vi "Main.vi"(8 "error in (no error)":errorcluster, 11 "DAQMH121119OrcaFlashBase in":refnum<class "DAQOrcaFlash.lvclass">) -> (0 "error out":errorcluster, 3 "component":refnum<class "DAQOrcaFlash.lvclass">)   [LabVIEW 2012, in "DAQOrcaFlash.lvclass"]
doc: "Main VI of the component."
uses:
  DAQOrcaFlash.lvclass
  binning.ctl
  visualisation_line_cluster.ctl
  merit_factor_type.ctl
  DAQOrcaFlash.lvclass/DAQOrcaFlash.ctl
  <vilib>/Distrio/Murmex/InitialiseMessage/InitialiseMessage.lvclass
  <vilib>/Distrio/Murmex/Murmex/command_enum.ctl
  <vilib>/Distrio/Murmex/TerminateMessage/TerminateMessage.lvclass
  <vilib>/Distrio/Murmex/StartMessage/StartMessage.lvclass
  <vilib>/Distrio/Murmex/StartMessage/run mode enum.ctl
  <vilib>/Distrio/Murmex/StopMessage/StopMessage.lvclass
  <vilib>/Distrio/Murmex/ConfigureMessage/ConfigureMessage.lvclass
  <vilib>/Distrio/Murmex/Murmex/update_cluster.ctl
  class variable.vi
  <vilib>/Distrio/Murmex/Murmex/Set VI reference.vi
  <vilib>/Distrio/Murmex/Murmex/Set configure at initialise.vi
  <vilib>/Distrio/Murmex/Murmex/Set relay start stop to observers.vi
  <vilib>/Distrio/Murmex/Murmex/Set log reference.vi
  <vilib>/Distrio/Murmex/Murmex/Set write log to disk.vi
  <vilib>/Distrio/Murmex/Murmex/Murmex.lvclass
  <vilib>/Distrio/Murmex/Message/Message.lvclass
panel:
  in  "button:configure":bool
  in  "button:quit":bool
  in  "terminate?":bool
  out "progress bar":sgl(slide) scale=0.0..1.0
  in  "Tab":T1(tab)
  in  "Rolling shutter pace":sgl[unit]=9.74436e-06 min=9.74436e-06 max=10 step=3.76e-09 format="%#_7g"
  out "Frames per second":dbl[unit]
  out "Virtual slit width":dbl[unit]
  in  "button:start_sweep":bool
  in  "y offset":u16 max=2048 step=4
  in  "x offset":u16 max=2048 step=4
  in  "y resolution":u16=2048 min=4 max=2048 step=4
  in  "x resolution":u16=2048 min=4 max=2048 step=4
  in  "binning":T2=1 items=["1x1"=1, "2x2"=2, "4x4"=4]
  in  "no. of frames":i32=1 min=1 step=1
  in  "line exposure time":dbl[unit]=0.1 caption="exposure time" min=9.700000000000001e-09 max=0.01
  in  "button:start focus":bool
  in  "file name":string
  in  "subfolder levels":string[](array[string])
  in  "Custom saving path":bool
  in  "directory out":path
  in  "button:convert":bool
  out "filename":string
  in  "directory in":path
  in  "ID":string="orca"
  in  "log":string
  out "time interval between MF":dbl
  out "Merit Factor":dbl
  in  "Merit factor type":T3
  in  "button:AO":bool
  in  "lines":T4[](array[typedef])
  in  "Conversion policy":T5={"Conversion Method"=10, "Minimum Value"=0, "Maximum Value"=0, "# Shifts"=0} {"Conversion Method" items=["Default"=10, "Most Significant Bits"=11, "Full Dynamic"=12, "Downshift"=13, "Given Range"=14, "90% Dynamic"=15, "Given Percent Range"=16]}
  # "Convert here properietary file formats of Hamamatsu to TIFF format."
  # "DAQOrcaFlash\n\nImplemented by:\nMarcel van 't Hoff\nLudovico Silvestri\nUniversity of Florence, Ital\n\nThis component supports only the Hamamatsu Orca Flash 4.0"
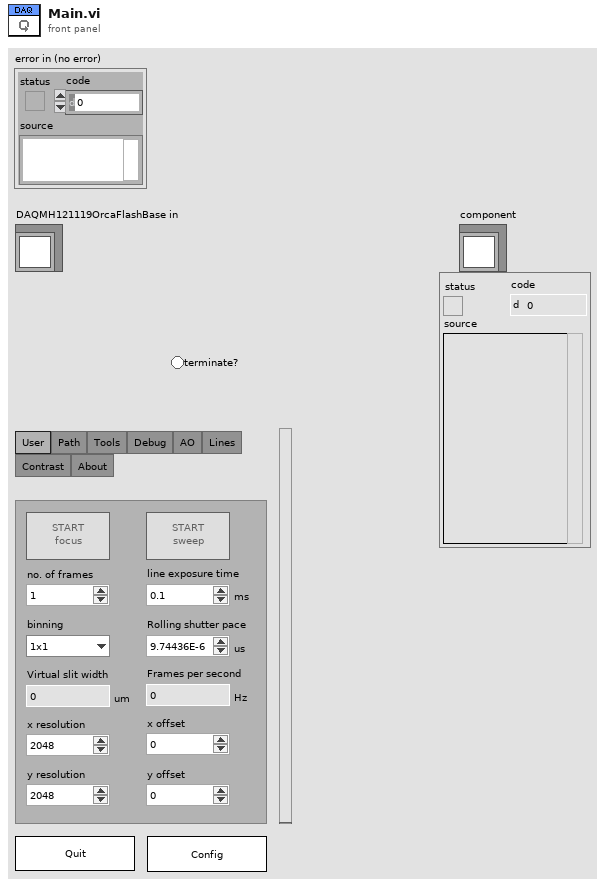
[diagram p1: front panel]
types:
  T1 = enum32{"User", "Path", "Tools", "Debug", "AO", "Lines", "Contrast", "About"}
  T2 = typedef "DAQOrcaFlash.lvclass/binning.ctl" = u16
  T3 = typedef "DAQOrcaFlash.lvclass/merit_factor_type.ctl" = enum16{"full frame intensity", "ROI beads", "Weber contrast", "Michelson contrast", "RMS contrast", "Line profile analysis", "ROI analysis", "FFT", "SNR", "5% brightest"}
  T4 = typedef "DAQOrcaFlash.lvclass/visualisation_line_cluster.ctl" = cluster{"direction":enum16{"horizontal", "vertical"}, "position":i32}
  T5 = cluster{"Conversion Method":u32, "Minimum Value":i32, "Maximum Value":i32, "# Shifts":i32}
  T6 = typedef "Murmex.lvlib/Murmex.lvclass/command_enum.ctl" = enum16{"null", "initialise", "reset", "terminate", "acknowledge", "update", "inspect", "inform", "proceed", "start", "stop", "fetch", "configure", "generic"}
  T7 = typedef "Murmex.lvlib/StartMessage.lvclass/run mode enum.ctl" = enum16{"infinite", "finite"}
  T8 = typedef "Murmex.lvlib/Murmex.lvclass/update_cluster.ctl" = cluster{"target ID":string, "key chains":string[], "values":variant[]}
  T9 = enum8{"Enabled", "Disabled", "Disabled and Grayed Out"}
  T10 = typedef "Murmex.lvclass/command_enum.ctl" = enum16{"null", "initialise", "reset", "terminate", "acknowledge", "update", "inspect", "inform", "proceed", "start", "stop", "fetch", "configure", "generic"}
  T11 = typedef "Murmex.lvclass/Event type enumerations.ctl" = enum16{"before", "after"}
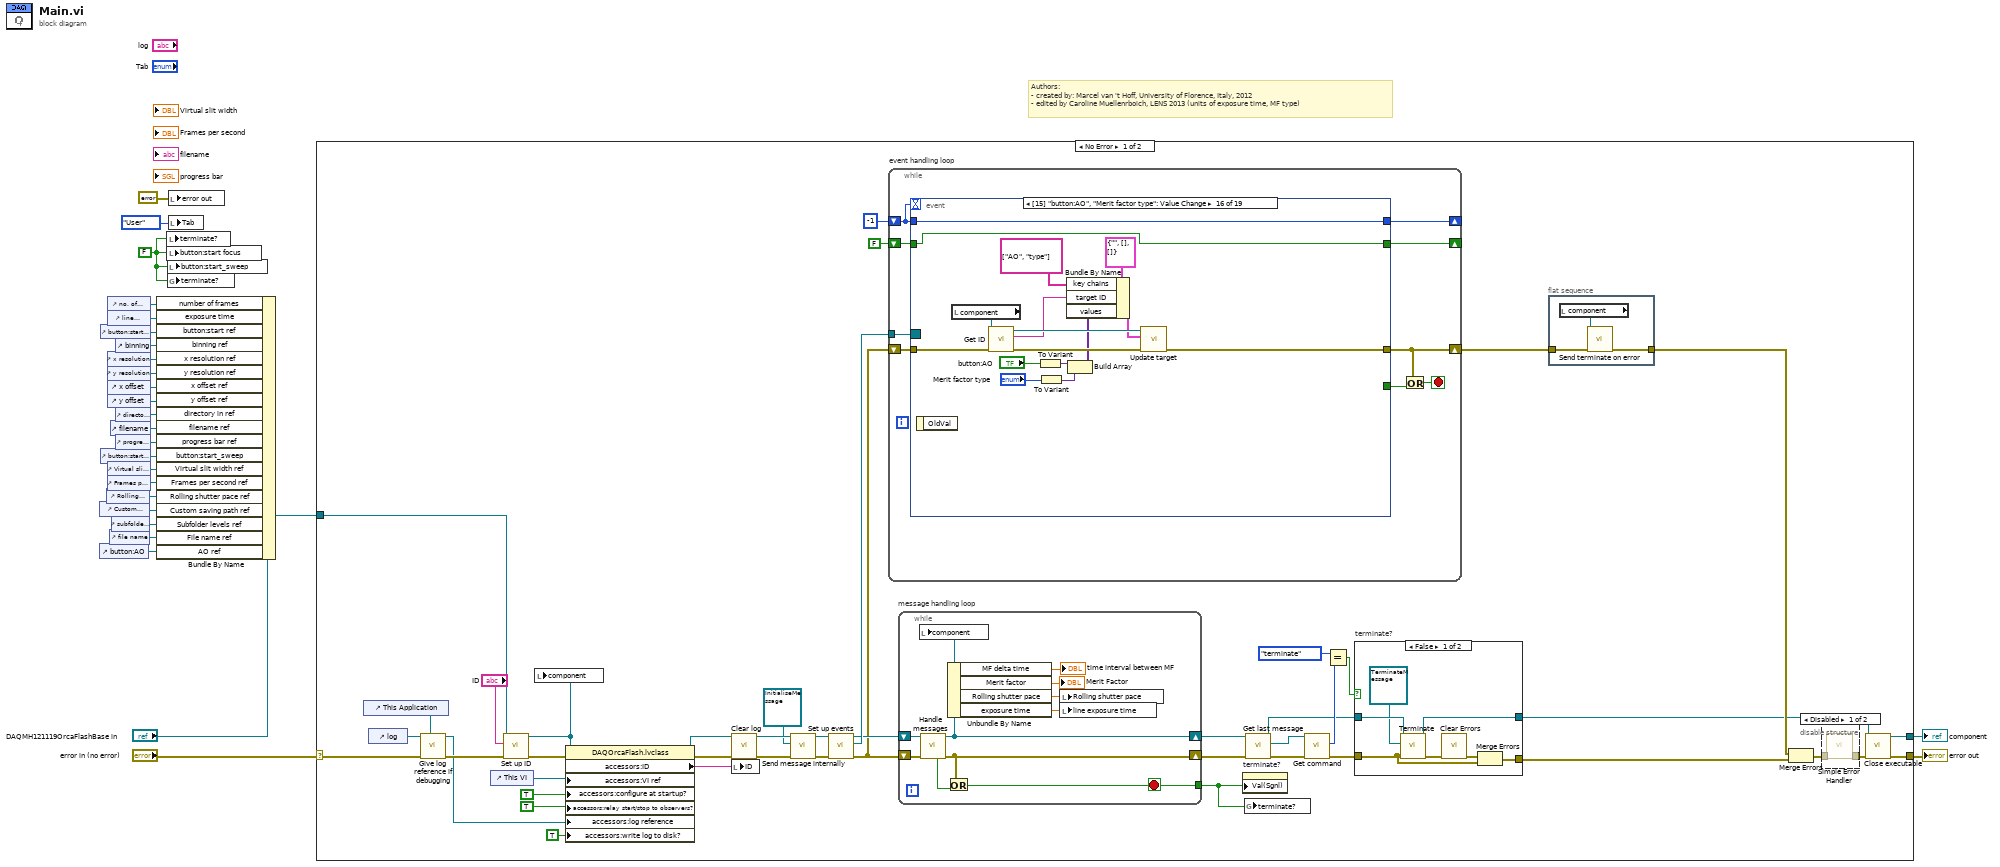
[diagram p0: block diagram]
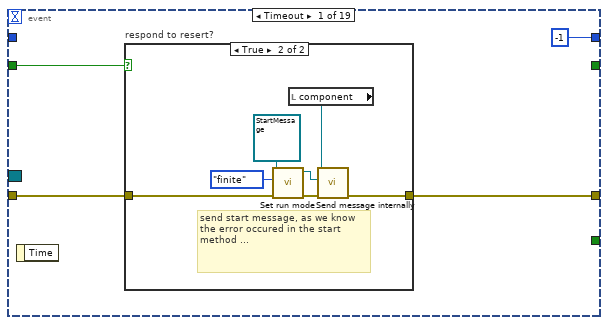
[diagram p4: hidden frame]
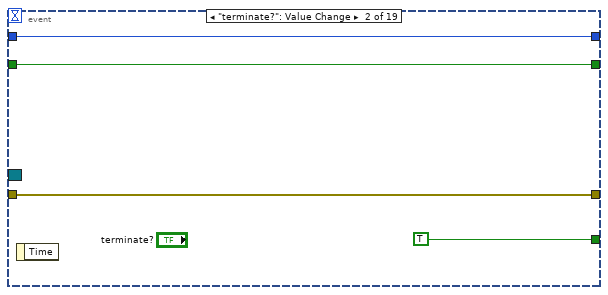
[diagram p6: hidden frame]
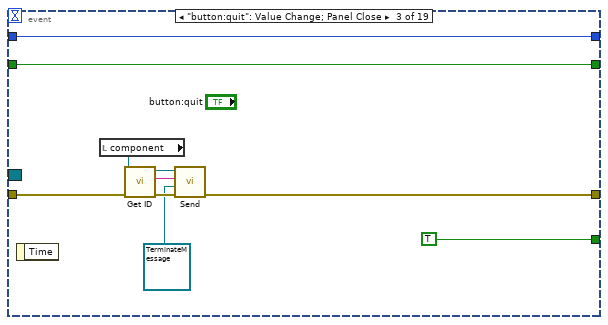
[diagram p7: hidden frame]
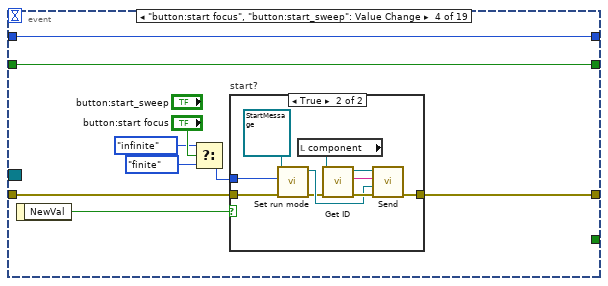
[diagram p8: hidden frame]
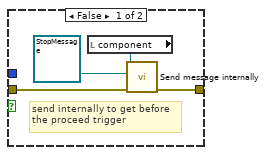
[diagram p9: hidden frame]
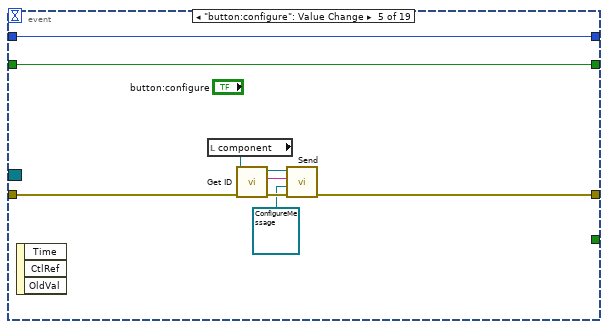
[diagram p10: hidden frame]
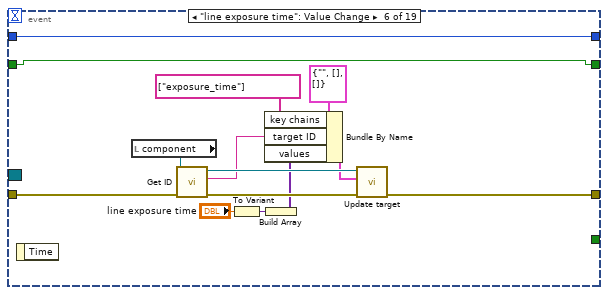
[diagram p11: hidden frame]
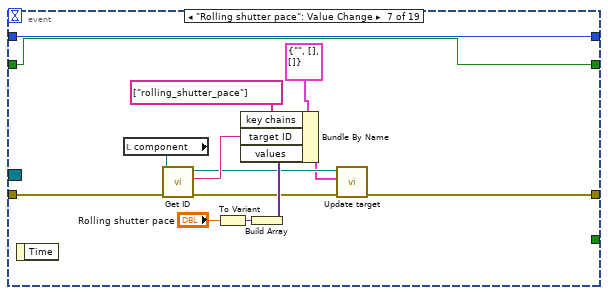
[diagram p12: hidden frame]
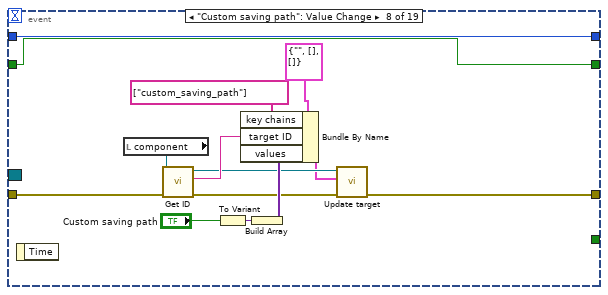
[diagram p13: hidden frame]
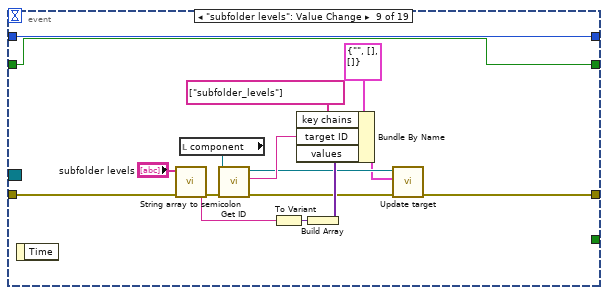
[diagram p14: hidden frame]
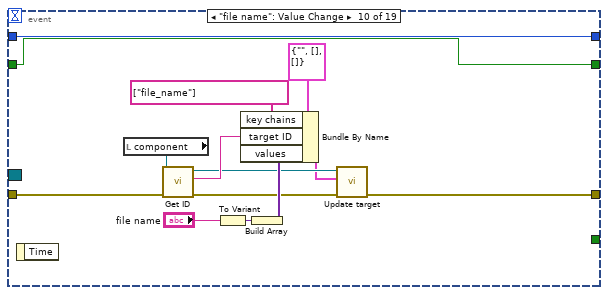
[diagram p15: hidden frame]
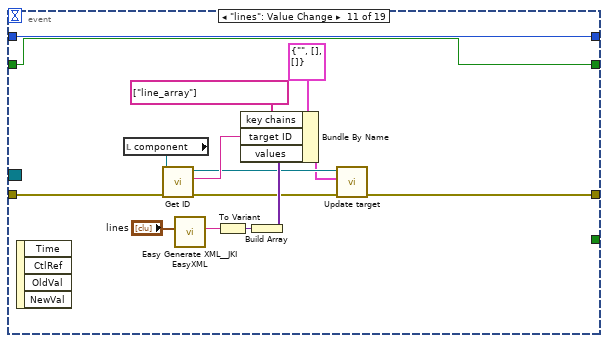
[diagram p16: hidden frame]
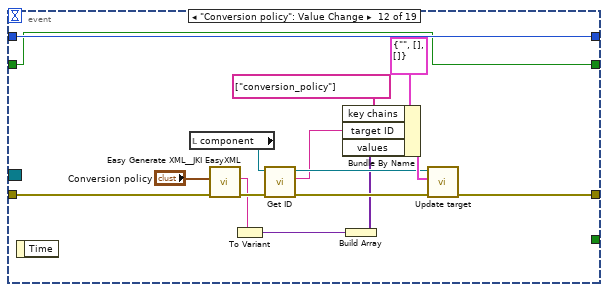
[diagram p17: hidden frame]
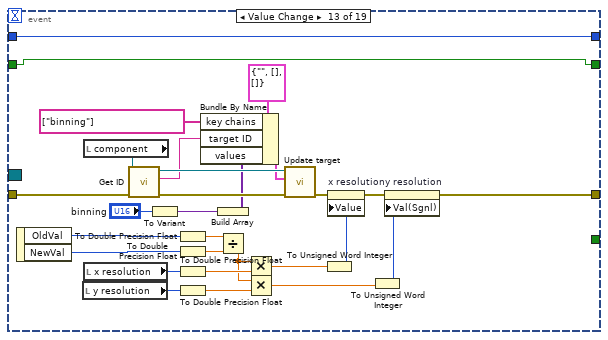
[diagram p18: hidden frame]
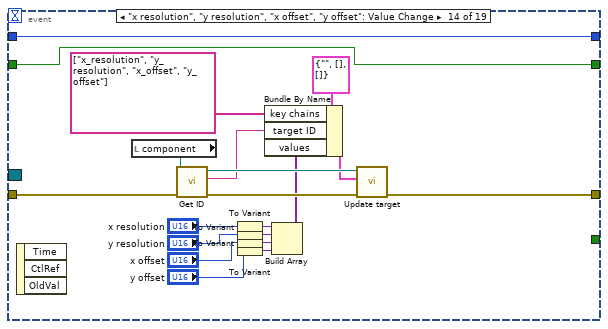
[diagram p19: hidden frame]
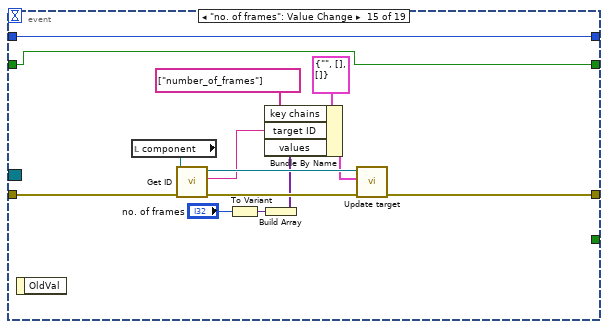
[diagram p20: hidden frame]
diagram:
  w9 = FALSE ("terminate?")
  # "Authors: \n- created by: Marcel van 't Hoff, University of Florence, Italy, 2012\n- edited by Caroline Muellenrboich, LENS 2013 (units of exposure time, MF type)"
  n1 = control-ref of="button:AO"() -> (w2:refnum<vi>)
  n2 = control-ref of="Custom saving path"() -> (w3:refnum<vi>)
  n3 = control-ref of="button:start focus"() -> (w20:refnum<vi>)
  n4 = control-ref of="button:start_sweep"() -> (w10:refnum<vi>)
  n5 = control-ref of="Rolling shutter pace"() -> (w6:refnum<vi>)
  n6 = control-ref of="no. of frames"() -> (w21:refnum<vi>)
  n7 = control-ref of="line exposure time"() -> (w22:refnum<vi>)
  n8 = control-ref of="x resolution"() -> (w18:refnum<vi>)
  n9 = control-ref of="y resolution"() -> (w17:refnum<vi>)
  n10 = control-ref of="x offset"() -> (w16:refnum<vi>)
  n11 = control-ref of="y offset"() -> (w15:refnum<vi>)
  n12 = control-ref of="Virtual slit width"() -> (w8:refnum<vi>)
  n13 = control-ref of="Frames per second"() -> (w7:refnum<vi>)
  n14 = control-ref of="file name"() -> (w5:refnum<vi>)
  n15 = control-ref of="filename"() -> (w13:refnum<vi>)
  n16 = control-ref of="subfolder levels"() -> (w4:refnum<vi>)
  n17 = control-ref of="binning"() -> (w19:refnum<vi>)
  n18 = control-ref of="directory in"() -> (w14:refnum<vi>)
  n19 = control-ref of="progress bar"() -> (w12:refnum<vi>)
  n20 = Bundle By Name(cluster="DAQMH121119OrcaFlashBase in", "number of frames"=w21, "exposure time"=w22, "button:start ref"=w20, "binning ref"=w19, "x resolution ref"=w18, "y resolution ref"=w17, "x offset ref"=w16, "y offset ref"=w15, "directory in ref"=w14, "filename ref"=w13, "progress bar ref"=w12, "button:start_sweep"=w10, "Virtual slit width ref"=w8, "Frames per second ref"=w7, "Rolling shutter pace ref"=w6, "Custom saving path ref"=w3, "Subfolder levels ref"=w4, "File name ref"=w5, "AO ref"=w2) -> (w23:refnum<class "DAQOrcaFlash.lvclass">)
  n21 = local write "terminate?"(w9) -> ()
  n22 = local write "button:start focus"(w9) -> ()
  n23 = local write "button:start_sweep"(w9) -> ()
  n24 = global write "class variable.vi" "terminate?"(w9) -> ()
  n25 = local write "error out"(errorcluster {"status"=FALSE, "code"=0, "source"=""} ("error out")) -> ()
  n26 = local write "Tab"(T1."User" ("Tab")) -> ()
  n27 = case shown="No Error" "error in (no error)" {
    selector: "error in (no error)" -> [w34 w423]
    tunnel: [w61 w423] -> w26
    tunnel: [w60 w422] -> w25
    tunnel: w23 -> [w66 w422]
    frame No Error {
      n28 = control-ref of="This Application"() -> (w30:refnum<vi>)
      n29 = control-ref of="log"() -> (w32:refnum<vi>)
      n30 = call "Give log reference if debugging.vi"("application ref"=w30, "error in (no error)"=w34, "log reference in"=w32) -> ("error out"=w33:errorcluster, "log reference out"=w31:refnum<vi>)  [unwired: 6 in, 1 out]
      n31 = control-ref of="This VI"() -> (w56:refnum<vi>)
      n32 = call <vilib>:"Set up ID.vi"("error in (no error)"=w33, "component ID"="ID", "MurmexBase in"=w66) -> ("error out"=w58:errorcluster, "MurmexBase out"=w47:refnum<class "DAQOrcaFlash.lvclass">)  [unwired: 6 in, 1 out]
      n33 = local write "component"(w47) -> ()
      n34 = property class="DAQOrcaFlash.lvclass"(reference=w47, error in=w58, "accessors:VI ref"=w56, "accessors:configure at startup?"=TRUE ("configure at startup?"), "accessors:relay start/stop to observers?"=TRUE ("relay start/stop to observers?"), "accessors:log reference"=w31, "accessors:write log to disk?"=TRUE ("write log to disk?")) -> (reference out=w54:refnum<class "DAQOrcaFlash.lvclass">, error out=w55:errorcluster, "accessors:ID"=w57:string)
      n35 = call <vilib>:"Clear log.vi"("error in (no error)"=w55, "MurmexBase in"=w54) -> ("error out"=w67:errorcluster, "MurmexBase out"=w71:refnum<class "DAQOrcaFlash.lvclass">)  [unwired: 8 in]
      n36 = local write "ID"(w57) -> ()
      n37 = call <vilib>:"Send message internally.vi"("error in (no error)"=w67, "Message"=refnum<class "InitialiseMessage.lvclass"> refnum ("Distrio Murmex 1.0:InitialiseMessage"), "Murmex in"=w71) -> ("error out"=w64:errorcluster, "Murmex out"=w63:refnum<class "DAQOrcaFlash.lvclass">)  [unwired: 7 in]
      n38 = call <vilib>:"Set up events.vi"("error in (no error)"=w64, "MurmexBase in"=w63) -> ("error out"=w36:errorcluster, "Event Registration Refnum"=w69:refnum<event-registration>, "MurmexBase out"=w38:refnum<class "DAQOrcaFlash.lvclass">)  [unwired: 7 in]
      n39 = while "event handling loop" {
        shift-right: [w95] -> _
        shift-left: -1 -> [w94]
        tunnel: w69 -> [w92]
        shift-right: [w91] -> w68
        shift-left: w36 -> [w93]
        shift-right: [w88] -> _
        shift-left: FALSE ("respond to reset?") -> [w87]
        stop <- w89 stop-if-true
        n40 = event shown="[15] \"button:AO\", \"Merit factor type\": Value Change" {
          selector: w92 -> [_ _ _ _ _ _ _ _ _ _ _ _ _ _ _ _ _ _ _]
          dyn-events: _ -> [_ _ _ _ _ _ _ _ _ _ _ _ _ _ _ _ _ _ _]
          timeout: w94 -> [_ _ _ _ _ _ _ _ _ _ _ _ _ _ _ _ _ _ _]
          tunnel: [-1 w111 w121 w130 w153 w167 w181 w195 w211 w225 w240 w256 w285 w305 w319 w335 w337 w399 w411] -> w95
          tunnel: w94 -> [_ w111 w121 w130 w153 w167 w181 w195 w211 w225 w240 w256 w285 w305 w319 w335 w342 w399 w411]
          tunnel: w93 -> [w97 w110 w114 w129 w149 w166 w180 w194 w200 w224 w239 w255 w284 w304 w318 w334 w343 w397 w408]
          tunnel: [w96 w110 w116 w128 w148 w165 w173 w183 w204 w217 w232 w250 w267 w303 w317 w323 w344 w396 w401] -> w91
          tunnel: [_ TRUE TRUE _ _ _ _ _ _ _ _ _ _ _ _ _ _ _ _] -> w90
          tunnel: [_ w108 w112 w122 w145 w154 w168 w182 w196 w212 w226 w241 w257 w286 w306 w322 w339 w393 w400] -> w88
          tunnel: w87 -> [w98 w108 w112 w122 w145 w154 w168 w182 w196 w212 w226 w241 w257 w286 w306 w322 w340 w393 w400]
          event Timeout {
            n41 = event-data() -> ()  [unwired: 1 in, 1 out]
            n42 = case "respond to resert?" shown="True" w98 {
              tunnel: w97 -> [w100 w103]
              tunnel: [w100 w107] -> w96
              frame False {
              }
              frame True {
                # "send start message, as we know the error occured in the start method ..."
                n43 = call <vilib>:"Set run mode.vi"("error in (no error)"=w103, "run mode"=run_mode_enum."finite", "StartMessage in"=refnum<class "StartMessage.lvclass"> refnum ("Distrio Murmex 1.0:StartMessage")) -> ("error out"=w102:errorcluster, "StartMessage out"=w104:refnum<class "StartMessage.lvclass">)  [unwired: 7 in]
                n44 = local read "component"() -> (w106:refnum<class "DAQOrcaFlash.lvclass">)
                n45 = call <vilib>:"Send message internally.vi"("error in (no error)"=w102, "Message"=w104, "Murmex in"=w106) -> ("error out"=w107:errorcluster)  [unwired: 7 in, 1 out]
              }
            }
          }
          event "terminate?": Value Change {
            n46 = event-data() -> ()  [unwired: 1 in, 1 out]
          }
          event "button:quit": Value Change; Panel Close {
            n47 = event-data() -> ()  [unwired: 1 in, 1 out]
            n48 = local read "component"() -> (w119:refnum<class "DAQOrcaFlash.lvclass">)
            n49 = call <vilib>:"Get ID.vi"("error in (no error)"=w114, "Murmex in"=w119) -> ("error out"=w115:errorcluster, "component id"=w117:string, "Murmex out"=w118:refnum<class "DAQOrcaFlash.lvclass">)  [unwired: 7 in]
            n50 = call <vilib>:"Send.vi"("error in (no error)"=w115, "Message"=refnum<class "TerminateMessage.lvclass"> refnum ("Message in"), "recipient"=w117, "Murmex in"=w118) -> ("error out"=w116:errorcluster)  [unwired: 6 in, 1 out]
          }
          event "button:start focus", "button:start_sweep": Value Change {
            n51 = event-data() -> ("NewVal"=w125:bool)  [unwired: 1 in]
            n52 = Select(t=run_mode_enum."infinite" ("run mode"), s="button:start focus", f=run_mode_enum."finite" ("run mode")) -> (s? t:f=w126:T7)
            n53 = case "start?" shown="True" w125 {
              tunnel: [w133 w140] -> w128
              tunnel: w129 -> [w134 w137]
              tunnel: w126 -> [_ w135]
              frame False {
                # "send internally to get before\nthe proceed trigger"
                n54 = local read "component"() -> (w132:refnum<class "DAQOrcaFlash.lvclass">)
                n55 = call <vilib>:"Send message internally.vi"("error in (no error)"=w134, "Message"=refnum<class "StopMessage.lvclass"> refnum ("Distrio Murmex 1.0:StopMessage"), "Murmex in"=w132) -> ("error out"=w133:errorcluster)  [unwired: 7 in, 1 out]
              }
              frame True {
                n56 = call <vilib>:"Set run mode.vi"("error in (no error)"=w137, "run mode"=w135, "StartMessage in"=refnum<class "StartMessage.lvclass"> refnum ("Distrio Murmex 1.0:StartMessage")) -> ("error out"=w136:errorcluster, "StartMessage out"=w138:refnum<class "StartMessage.lvclass">)  [unwired: 7 in]
                n57 = local read "component"() -> (w144:refnum<class "DAQOrcaFlash.lvclass">)
                n58 = call <vilib>:"Get ID.vi"("error in (no error)"=w136, "Murmex in"=w144) -> ("error out"=w141:errorcluster, "component id"=w142:string, "Murmex out"=w143:refnum<class "DAQOrcaFlash.lvclass">)  [unwired: 7 in]
                n59 = call <vilib>:"Send.vi"("error in (no error)"=w141, "Message"=w138, "recipient"=w142, "Murmex in"=w143) -> ("error out"=w140:errorcluster)  [unwired: 6 in, 1 out]
              }
            }
          }
          event "button:configure": Value Change {
            n60 = event-data() -> ()  [unwired: 1 in, 3 out]
            n61 = local read "component"() -> (w147:refnum<class "DAQOrcaFlash.lvclass">)
            n62 = call <vilib>:"Get ID.vi"("error in (no error)"=w149, "Murmex in"=w147) -> ("error out"=w150:errorcluster, "component id"=w151:string, "Murmex out"=w152:refnum<class "DAQOrcaFlash.lvclass">)  [unwired: 7 in]
            n63 = call <vilib>:"Send.vi"("error in (no error)"=w150, "Message"=refnum<class "ConfigureMessage.lvclass"> refnum ("ConfigureMessage"), "recipient"=w151, "Murmex in"=w152) -> ("error out"=w148:errorcluster)  [unwired: 6 in, 1 out]
          }
          event "line exposure time": Value Change {
            n64 = event-data() -> ()  [unwired: 1 in, 1 out]
            n65 = local read "component"() -> (w164:refnum<class "DAQOrcaFlash.lvclass">)
            n66 = call <vilib>:"Get ID.vi"("error in (no error)"=w166, "Murmex in"=w164) -> ("error out"=w162:errorcluster, "component id"=w159:string, "Murmex out"=w163:refnum<class "DAQOrcaFlash.lvclass">)  [unwired: 7 in]
            n67 = To Variant(anything="line exposure time") -> (Variant=w157:variant)
            n68 = Build Array(w157) -> (w156:variant[])
            n69 = Bundle By Name(cluster=T8 {"target ID"="", "key chains"=[], "values"=[]} ("update cluster"), "key chains"=string[] ["exposure_time"], "target ID"=w159, "values"=w156) -> (w160:T8)
            n70 = call <vilib>:"Update target.vi"("error in (no error)"=w162, "update cluster"=w160, "MurmexBase in"=w163) -> ("error out"=w165:errorcluster)  [unwired: 7 in, 1 out]
          }
          event "Rolling shutter pace": Value Change {
            n71 = event-data() -> ()  [unwired: 1 in, 1 out]
            n72 = local read "component"() -> (w178:refnum<class "DAQOrcaFlash.lvclass">)
            n73 = call <vilib>:"Get ID.vi"("error in (no error)"=w180, "Murmex in"=w178) -> ("error out"=w174:errorcluster, "component id"=w177:string, "Murmex out"=w172:refnum<class "DAQOrcaFlash.lvclass">)  [unwired: 7 in]
            n74 = To Variant(anything="Rolling shutter pace") -> (Variant=w179:variant)
            n75 = Build Array(w179) -> (w175:variant[])
            n76 = Bundle By Name(cluster=T8 {"target ID"="", "key chains"=[], "values"=[]} ("update cluster"), "key chains"=string[] ["rolling_shutter_pace"], "target ID"=w177, "values"=w175) -> (w170:T8)
            n77 = call <vilib>:"Update target.vi"("error in (no error)"=w174, "update cluster"=w170, "MurmexBase in"=w172) -> ("error out"=w173:errorcluster)  [unwired: 7 in, 1 out]
          }
          event "Custom saving path": Value Change {
            n78 = event-data() -> ()  [unwired: 1 in, 1 out]
            n79 = local read "component"() -> (w192:refnum<class "DAQOrcaFlash.lvclass">)
            n80 = call <vilib>:"Get ID.vi"("error in (no error)"=w194, "Murmex in"=w192) -> ("error out"=w188:errorcluster, "component id"=w191:string, "Murmex out"=w187:refnum<class "DAQOrcaFlash.lvclass">)  [unwired: 7 in]
            n81 = To Variant(anything="Custom saving path") -> (Variant=w193:variant)
            n82 = Build Array(w193) -> (w189:variant[])
            n83 = Bundle By Name(cluster=T8 {"target ID"="", "key chains"=[], "values"=[]} ("update cluster"), "key chains"=string[] ["custom_saving_path"], "target ID"=w191, "values"=w189) -> (w185:T8)
            n84 = call <vilib>:"Update target.vi"("error in (no error)"=w188, "update cluster"=w185, "MurmexBase in"=w187) -> ("error out"=w183:errorcluster)  [unwired: 7 in, 1 out]
          }
          event "subfolder levels": Value Change {
            n85 = event-data() -> ()  [unwired: 1 in, 1 out]
            n86 = call "String array to semicolon.vi"("error in"=w200, "String array"="subfolder levels") -> ("error out"=w199:errorcluster, "Semicolon string"=w198:string)  [unwired: 8 in]
            n87 = local read "component"() -> (w209:refnum<class "DAQOrcaFlash.lvclass">)
            n88 = call <vilib>:"Get ID.vi"("error in (no error)"=w199, "Murmex in"=w209) -> ("error out"=w205:errorcluster, "component id"=w208:string, "Murmex out"=w203:refnum<class "DAQOrcaFlash.lvclass">)  [unwired: 7 in]
            n89 = To Variant(anything=w198) -> (Variant=w210:variant)
            n90 = Build Array(w210) -> (w206:variant[])
            n91 = Bundle By Name(cluster=T8 {"target ID"="", "key chains"=[], "values"=[]} ("update cluster"), "key chains"=string[] ["subfolder_levels"], "target ID"=w208, "values"=w206) -> (w201:T8)
            n92 = call <vilib>:"Update target.vi"("error in (no error)"=w205, "update cluster"=w201, "MurmexBase in"=w203) -> ("error out"=w204:errorcluster)  [unwired: 7 in, 1 out]
          }
          event "file name": Value Change {
            n93 = event-data() -> ()  [unwired: 1 in, 1 out]
            n94 = local read "component"() -> (w222:refnum<class "DAQOrcaFlash.lvclass">)
            n95 = call <vilib>:"Get ID.vi"("error in (no error)"=w224, "Murmex in"=w222) -> ("error out"=w218:errorcluster, "component id"=w221:string, "Murmex out"=w216:refnum<class "DAQOrcaFlash.lvclass">)  [unwired: 7 in]
            n96 = To Variant(anything="file name") -> (Variant=w223:variant)
            n97 = Build Array(w223) -> (w219:variant[])
            n98 = Bundle By Name(cluster=T8 {"target ID"="", "key chains"=[], "values"=[]} ("update cluster"), "key chains"=string[] ["file_name"], "target ID"=w221, "values"=w219) -> (w214:T8)
            n99 = call <vilib>:"Update target.vi"("error in (no error)"=w218, "update cluster"=w214, "MurmexBase in"=w216) -> ("error out"=w217:errorcluster)  [unwired: 7 in, 1 out]
          }
          event "lines": Value Change {
            n100 = event-data() -> ()  [unwired: 1 in, 4 out]
            n101 = local read "component"() -> (w237:refnum<class "DAQOrcaFlash.lvclass">)
            n102 = call <vilib>:"Get ID.vi"("error in (no error)"=w239, "Murmex in"=w237) -> ("error out"=w233:errorcluster, "component id"=w236:string, "Murmex out"=w231:refnum<class "DAQOrcaFlash.lvclass">)  [unwired: 7 in]
            n103 = call <vilib>:"Easy Generate XML__JKI EasyXML.vi"("LabVIEW Data"="lines") -> ("XML String"=w227:string)  [unwired: 9 in, 1 out]
            n104 = To Variant(anything=w227) -> (Variant=w238:variant)
            n105 = Build Array(w238) -> (w234:variant[])
            n106 = Bundle By Name(cluster=T8 {"target ID"="", "key chains"=[], "values"=[]} ("update cluster"), "key chains"=string[] ["line_array"], "target ID"=w236, "values"=w234) -> (w229:T8)
            n107 = call <vilib>:"Update target.vi"("error in (no error)"=w233, "update cluster"=w229, "MurmexBase in"=w231) -> ("error out"=w232:errorcluster)  [unwired: 7 in, 1 out]
          }
          event "Conversion policy": Value Change {
            n108 = event-data() -> ()  [unwired: 1 in, 1 out]
            n109 = local read "component"() -> (w251:refnum<class "DAQOrcaFlash.lvclass">)
            n110 = call <vilib>:"Easy Generate XML__JKI EasyXML.vi"("error in (no error)"=w255, "LabVIEW Data"="Conversion policy") -> ("error out"=w254:errorcluster, "XML String"=w243:string)  [unwired: 8 in]
            n111 = To Variant(anything=w243) -> (Variant=w244:variant)
            n112 = call <vilib>:"Get ID.vi"("error in (no error)"=w254, "Murmex in"=w251) -> ("error out"=w252:errorcluster, "component id"=w245:string, "Murmex out"=w246:refnum<class "DAQOrcaFlash.lvclass">)  [unwired: 7 in]
            n113 = Build Array(w244) -> (w242:variant[])
            n114 = Bundle By Name(cluster=T8 {"target ID"="", "key chains"=[], "values"=[]} ("update cluster"), "key chains"=string[] ["conversion_policy"], "target ID"=w245, "values"=w242) -> (w247:T8)
            n115 = call <vilib>:"Update target.vi"("error in (no error)"=w252, "update cluster"=w247, "MurmexBase in"=w246) -> ("error out"=w250:errorcluster)  [unwired: 7 in, 1 out]
          }
          event Value Change {
            n116 = event-data() -> ("OldVal"=w262:T2, "NewVal"=w261:T2)  [unwired: 1 in]
            n117 = local read "y resolution"() -> (w275:u16)
            n118 = local read "component"() -> (w283:refnum<class "DAQOrcaFlash.lvclass">)
            n119 = local read "x resolution"() -> (w274:u16)
            n120 = call <vilib>:"Get ID.vi"("error in (no error)"=w284, "Murmex in"=w283) -> ("error out"=w281:errorcluster, "component id"=w278:string, "Murmex out"=w282:refnum<class "DAQOrcaFlash.lvclass">)  [unwired: 7 in]
            n121 = To Variant(anything="binning") -> (Variant=w270:variant)
            n122 = To Double Precision Float(number=w262) -> (double precision float=w260:dbl)
            n123 = To Double Precision Float(number=w261) -> (double precision float=w259:dbl)
            n124 = To Double Precision Float(number=w274) -> (double precision float=w271:dbl)
            n125 = To Double Precision Float(number=w275) -> (double precision float=w272:dbl)
            n126 = Build Array(w270) -> (w276:variant[])
            n127 = Bundle By Name(cluster=T8 {"target ID"="", "key chains"=[], "values"=[]} ("update cluster"), "key chains"=string[] ["binning"], "target ID"=w278, "values"=w276) -> (w279:T8)
            n128 = Divide(x=w260, y=w259) -> (x/y=w258:dbl)
            n129 = Multiply(x=w258, y=w271) -> (x*y=w268:dbl)
            n130 = Multiply(x=w258, y=w272) -> (x*y=w269:dbl)
            n131 = call <vilib>:"Update target.vi"("error in (no error)"=w281, "update cluster"=w279, "MurmexBase in"=w282) -> ("error out"=w266:errorcluster)  [unwired: 7 in, 1 out]
            n132 = To Unsigned Word Integer(number=w268) -> (unsigned 16bit integer=w265:u16)
            n133 = property on="x resolution" class="DigNum (strict)"(error in=w266, "Value"=w265) -> (error out=w263:errorcluster)  [unwired: 1 in, 1 out]
            n134 = To Unsigned Word Integer(number=w269) -> (unsigned 16bit integer=w264:u16)
            n135 = property on="y resolution" class="DigNum (strict)"(error in=w263, "Val(Sgnl)"=w264) -> (error out=w267:errorcluster)  [unwired: 1 in, 1 out]
          }
          event "x resolution", "y resolution", "x offset", "y offset": Value Change {
            n136 = event-data() -> ()  [unwired: 1 in, 3 out]
            n137 = local read "component"() -> (w302:refnum<class "DAQOrcaFlash.lvclass">)
            n138 = call <vilib>:"Get ID.vi"("error in (no error)"=w304, "Murmex in"=w302) -> ("error out"=w300:errorcluster, "component id"=w297:string, "Murmex out"=w301:refnum<class "DAQOrcaFlash.lvclass">)  [unwired: 7 in]
            n139 = To Variant(anything="x resolution") -> (Variant=w290:variant)
            n140 = To Variant(anything="y resolution") -> (Variant=w289:variant)
            n141 = To Variant(anything="x offset") -> (Variant=w288:variant)
            n142 = To Variant(anything="y offset") -> (Variant=w287:variant)
            n143 = Build Array(w290, w289, w288, w287) -> (w291:variant[])
            n144 = Bundle By Name(cluster=T8 {"target ID"="", "key chains"=[], "values"=[]} ("update cluster"), "key chains"=string[] ["x_resolution", "y_resolution", "x_offset", "y_offset"], "target ID"=w297, "values"=w291) -> (w298:T8)
            n145 = call <vilib>:"Update target.vi"("error in (no error)"=w300, "update cluster"=w298, "MurmexBase in"=w301) -> ("error out"=w303:errorcluster)  [unwired: 7 in, 1 out]
          }
          event "no. of frames": Value Change {
            n146 = event-data() -> ()  [unwired: 1 in, 1 out]
            n147 = local read "component"() -> (w316:refnum<class "DAQOrcaFlash.lvclass">)
            n148 = call <vilib>:"Get ID.vi"("error in (no error)"=w318, "Murmex in"=w316) -> ("error out"=w314:errorcluster, "component id"=w311:string, "Murmex out"=w315:refnum<class "DAQOrcaFlash.lvclass">)  [unwired: 7 in]
            n149 = To Variant(anything="no. of frames") -> (Variant=w307:variant)
            n150 = Build Array(w307) -> (w309:variant[])
            n151 = Bundle By Name(cluster=T8 {"target ID"="", "key chains"=[], "values"=[]} ("update cluster"), "key chains"=string[] ["number_of_frames"], "target ID"=w311, "values"=w309) -> (w312:T8)
            n152 = call <vilib>:"Update target.vi"("error in (no error)"=w314, "update cluster"=w312, "MurmexBase in"=w315) -> ("error out"=w317:errorcluster)  [unwired: 7 in, 1 out]
          }
          event "button:AO": Value Change {
            n153 = event-data() -> ()  [unwired: 1 in, 1 out]
            n154 = local read "component"() -> (w333:refnum<class "DAQOrcaFlash.lvclass">)
            n155 = call <vilib>:"Get ID.vi"("error in (no error)"=w334, "Murmex in"=w333) -> ("error out"=w331:errorcluster, "component id"=w324:string, "Murmex out"=w332:refnum<class "DAQOrcaFlash.lvclass">)  [unwired: 7 in]
            n156 = To Variant(anything="button:AO") -> (Variant=w326:variant)
            n157 = To Variant(anything="Merit factor type") -> (Variant=w321:variant)
            n158 = Build Array(w326, w321) -> (w327:variant[])
            n159 = Bundle By Name(cluster=T8 {"target ID"="", "key chains"=[], "values"=[]} ("update cluster"), "key chains"=string[] ["AO", "type"], "target ID"=w324, "values"=w327) -> (w329:T8)
            n160 = call <vilib>:"Update target.vi"("error in (no error)"=w331, "update cluster"=w329, "MurmexBase in"=w332) -> ("error out"=w323:errorcluster)  [unwired: 7 in, 1 out]
          }
          event User Event {
            w336 = 5000  # wait for starting
            n161 = event-data() -> ("command"=w345:T10, "event type"=w341:T11)  [unwired: 1 in]
            n162 = case "command?" shown="\"reset\"" w345 {
              tunnel: [w350 w362 w374 w389 w392] -> w344
              tunnel: w343 -> [w349 w361 w375 w389 w392]
              tunnel: [w348 w360 w373 w387 w391] -> w338
              tunnel: w342 -> [w348 w360 w372 w387 w391]
              tunnel: w341 -> [w347 w359 w371 _ _]
              tunnel: [w346 w358 w370 w388 w390] -> w339
              tunnel: w340 -> [w346 w358 w370 _ w390]
              frame "stop" {
                n163 = case shown="\"after\"" w347 {
                  tunnel: [w351 w357] -> w350
                  tunnel: w349 -> [w351 w354]
                  frame "before", Default {
                  }
                  frame "after" {
                    n164 = local read "component"() -> (w355:refnum<class "DAQOrcaFlash.lvclass">)
                    n165 = call "Get GUI refs.vi"("error in (no error)"=w354, "DAQMH121119OrcaFlash in"=w355) -> ("error out"=w353:errorcluster, "Array"=w352:refnum<vi>[])  [unwired: 7 in, 1 out]
                    n166 = call <vilib>:"Disable GUI elements.vi"("error in (no error)"=w353, "enabled state"=T9."Enabled", "control refs"=w352) -> ("error out"=w357:errorcluster)  [unwired: 8 in]
                  }
                }
              }
              frame "start" {
                n167 = case shown="\"after\"" w359 {
                  tunnel: [w363 w369] -> w362
                  tunnel: w361 -> [w363 w367]
                  frame "before", Default {
                  }
                  frame "after" {
                    n168 = local read "component"() -> (w364:refnum<class "DAQOrcaFlash.lvclass">)
                    n169 = call "Get GUI refs.vi"("error in (no error)"=w367, "DAQMH121119OrcaFlash in"=w364) -> ("error out"=w366:errorcluster, "Array"=w365:refnum<vi>[])  [unwired: 7 in, 1 out]
                    n170 = call <vilib>:"Disable GUI elements.vi"("error in (no error)"=w366, "enabled state"=T9."Disabled and Grayed Out", "control refs"=w365) -> ("error out"=w369:errorcluster)  [unwired: 8 in]
                  }
                }
              }
              frame "initialise" {
                n171 = case shown="\"before\", Default" w371 {
                  tunnel: w375 -> [w377 w385]
                  tunnel: [w376 w384] -> w374
                  tunnel: [w382 -1] -> w373
                  tunnel: w372 -> [w382 _]
                  frame "before", Default {
                    n172 = local read "component"() -> (w378:refnum<class "DAQOrcaFlash.lvclass">)
                    n173 = call "Get GUI refs.vi"("error in (no error)"=w377, "DAQMH121119OrcaFlash in"=w378) -> ("error out"=w380:errorcluster, "Array"=w379:refnum<vi>[])  [unwired: 7 in, 1 out]
                    n174 = call <vilib>:"Disable GUI elements.vi"("error in (no error)"=w380, "enabled state"=T9."Disabled and Grayed Out", "control refs"=w379) -> ("error out"=w376:errorcluster)  [unwired: 8 in]
                  }
                  frame "after" {
                    n175 = local read "component"() -> (w386:refnum<class "DAQOrcaFlash.lvclass">)
                    n176 = call "Initialise parameters.vi"("error in (no error)"=w385, "DAQMH121119OrcaFlash in"=w386) -> ("error out"=w384:errorcluster)  [unwired: 8 in, 1 out]
                  }
                }
              }
              frame "reset" {
                w388 = TRUE  # respond to reset?
              }
              frame Default {
              }
            }
            n177 = Select(t=w336, s=w339, f=w338) -> (s? t:f=w337:i32)
          }
          event "button:convert": Value Change {
            n178 = event-data() -> ()  [unwired: 1 in, 1 out]
            n179 = local read "component"() -> (w398:refnum<class "DAQOrcaFlash.lvclass">)
            n180 = call "Convert directory new.vi"("error in (no error)"=w397, "directory out"="directory out", "directory in"="directory in", "DAQOrcaFlash in"=w398) -> ("error out"=w396:errorcluster)  [unwired: 6 in, 1 out]
          }
          event "directory in", "directory out": Value Change {
            n181 = event-data() -> ()  [unwired: 1 in, 1 out]
            n182 = local read "directory out"() -> (w410:path)
            n183 = local read "directory in"() -> (w407:path)
            n184 = call <vilib>:"Check if File or Folder Exists.vi"("error in (no error)"=w408, "path"=w410) -> ("error out"=w409:errorcluster, "file or folder exists?"=w405:bool)  [unwired: 7 in, 1 out]
            n185 = call <vilib>:"Check if File or Folder Exists.vi"("error in (no error)"=w409, "path"=w407) -> ("error out"=w402:errorcluster, "file or folder exists?"=w406:bool)  [unwired: 7 in, 1 out]
            n186 = And(x=w406, y=w405) -> (x .and. y?=w404:bool)
            n187 = call "bool_to_enable_state.vi"("boolean in"=w404) -> ("enabled status out"=w403:T9)  [unwired: 4 in]
            n188 = property on="button:convert" class="Bool"(error in=w402, "DisabledEnum"=w403) -> (error out=w401:errorcluster)  [unwired: 1 in, 1 out]
          }
        }
        n189 = Or(x=w91, y=w90) -> (x .or. y?=w89:bool)
      }
      n190 = while "message handling loop" {
        shift-right: [w417] -> w44
        shift-left: w36 -> [w419]
        shift-right: [w416] -> w46
        shift-left: w38 -> [w421]
        tunnel: [w418] -> w37
        stop <- w418 stop-if-true
        n191 = call <vilib>:"Handle messages.vi"("error in (no error)"=w419, "Murmex in"=w421) -> ("error out"=w417:errorcluster, "Murmex out"=w416:refnum<class "DAQOrcaFlash.lvclass">, "terminated?"=w420:bool)  [unwired: 7 in]
        n192 = local write "component"(w416) -> ()
        n193 = Or(x=w417, y=w420) -> (x .or. y?=w418:bool)
        n194 = Unbundle By Name(w416) -> ("MF delta time"=→"time interval between MF":dbl, "Merit factor"=→"Merit Factor":dbl, "Rolling shutter pace"=w415:sgl[unit], "exposure time"=w414:dbl[unit])
        n195 = local write "Rolling shutter pace"(w415) -> ()
        n196 = local write "line exposure time"(w414) -> ()
      }
      n197 = property on="terminate?" class="Bool (strict)"("Val(Sgnl)"=w37) -> ()  [unwired: 2 in, 2 out]
      n198 = global write "class variable.vi" "terminate?"(w37) -> ()
      n199 = call <vilib>:"Get last message.vi"("error in (no error)"=w44, "MurmexBase in"=w46) -> ("error out"=w43:errorcluster, "Message"=w42:refnum<class "Message.lvclass">, "MurmexBase out"=w45:refnum<class "DAQOrcaFlash.lvclass">)  [unwired: 7 in]
      n200 = call <vilib>:"Get command.vi"("error in (no error)"=w43, "Message in"=w42) -> ("error out"=w50:errorcluster, "command"=w52:T6)  [unwired: 7 in, 1 out]
      n201 = Equal?(x=command_enum."terminate", y=w52) -> (x = y?=w48:bool)
      n202 = case "terminate?" shown="False" w48 {
        tunnel: w45 -> [w80 w83]
        tunnel: [w79 w83] -> w59
        tunnel: w50 -> [w78 w82]
        tunnel: [w76 w82] -> w49
        frame False {
          n203 = call-dynamic "Terminate.vi"("error in (no error)"=w78, "Message in"=refnum<class "TerminateMessage.lvclass"> refnum, "DAQMH121119OrcaFlash in"=w80) -> ("error out"=w81:errorcluster, "DAQMH121119OrcaFlash out"=w79:refnum<class "DAQOrcaFlash.lvclass">)  [unwired: 7 in]
          n204 = call <vilib>:"Clear Errors.vi"("error in (no error)"=w81) -> ("error out"=w77:errorcluster)  [unwired: 6 in]
          n205 = Merge Errors(w77, w78) -> (w76:errorcluster)
        }
        frame True {
        }
      }
      n206 = flat-sequence {
        tunnel: w68 -> [w86]
        tunnel: [w84] -> w62
        frame #0 {
          n207 = local read "component"() -> (w85:refnum<class "DAQOrcaFlash.lvclass">)
          n208 = call <vilib>:"Send terminate on error.vi"("error in (no error)"=w86, "Murmex in"=w85) -> ("error out"=w84:errorcluster)  [unwired: 8 in, 1 out]
        }
      }
      n209 = Merge Errors(w62, w49) -> (w40:errorcluster)
      n210 = disable-structure shown="Disabled" {
        disable-tunnel: w40 -> [w73 w74]
        disable-tunnel: [w72 w74] -> w39
        frame Disabled {
          n211 = call <vilib>:"Simple Error Handler.vi"("error in (no error)"=w73) -> ("error out"=w72:errorcluster)  [unwired: 4 in, 4 out]
        }
        frame Enabled {
        }
      }
      n212 = call <vilib>:"Close executable.vi"("error in (no error)"=w39, "MurmexBase in"=w59) -> ("error out"=w61:errorcluster, "MurmexBase out"=w60:refnum<class "DAQOrcaFlash.lvclass">)  [unwired: 8 in]
    }
    frame Error {
    }
  }
  "error out" <- w26
  "component" <- w25
